vi "Set Column Width.vi"(7 "Sheet Name":string, 8 "error in":errorcluster, 9 "Width":dbl=8.43, 10 "Columns Range":string="A:C", 11 "SpreadsheetDoc":refnum<k24>) -> (0 "error out":errorcluster, 3 "SpreadsheetDoc out":refnum<k24>)   [LabVIEW 2019, in "Open Xml.lvlib"]
uses:
  Open Xml.lvlib
  D:/git/Open-Xml-LabVIEW/Source/DocumentFormat.OpenXml.dll
  DocumentFormat.OpenXml.dll
  D:/git/Open-Xml-LabVIEW/Source/DocumentFormat.OpenXml.Framework.dll
  DocumentFormat.OpenXml.Framework.dll
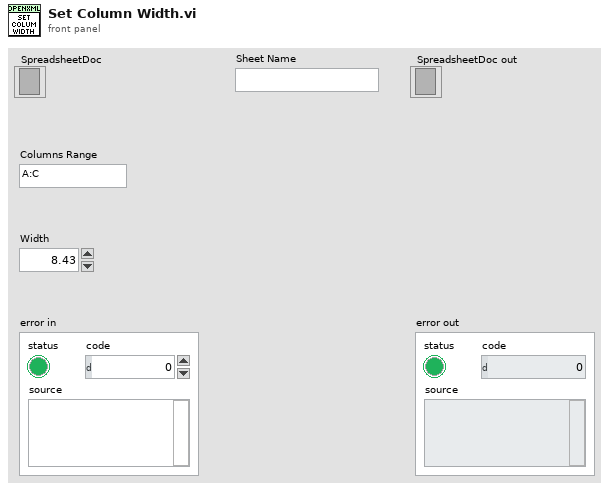
[diagram p1: front panel]
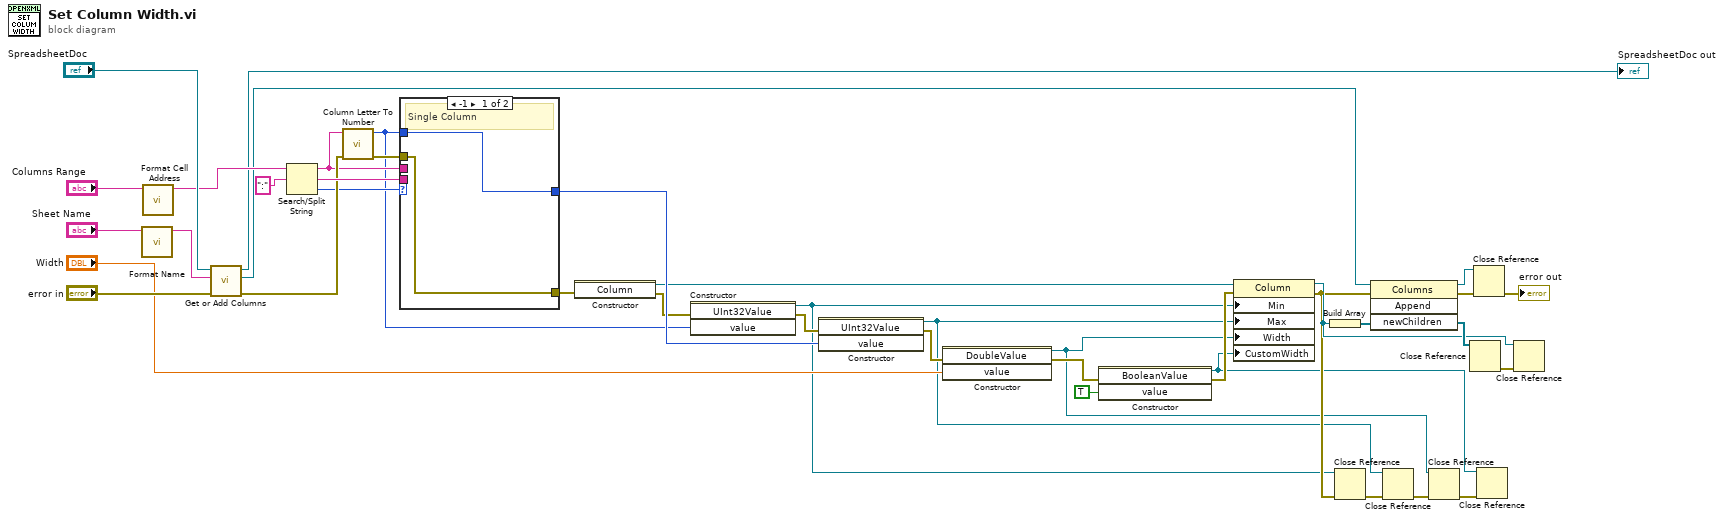
[diagram p0: block diagram]
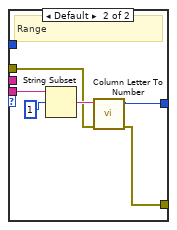
[diagram p2: hidden frame]
diagram:
  n1 = call "Format Name.vi"("Sheet Name"="Sheet Name") -> ("Formatted Sheet Name"=w37:string)  [unwired: 10 in]
  n2 = call "Format Cell Address.vi"("Cell Address"="Columns Range") -> ("Formatted Cell Address"=w35:string)  [unwired: 10 in]
  n3 = call "Get or Add Columns.vi"("error in"="error in", "Sheet Name"=w37, "SpreadsheetDoc in"="SpreadsheetDoc") -> ("error out"=w32:errorcluster, "Columns"=w17:refnum<k24>, "SpreadsheetDoc out"=→"SpreadsheetDoc out":refnum<k24>)  [unwired: 6 in]
  n4 = Search/Split String(string=w35, search string/char (-)=":") -> (substring before match=w29:string, match + rest of string=w33:string, offset of match=w31:i32)  [unwired: 1 in]
  n5 = call "Column Letter To Number.vi"("error in"=w32, "Letter"=w29) -> ("error out"=w30:errorcluster, "Number"=w18:i32)  [unwired: 8 in]
  n6 = case shown="-1" w31 {
    tunnel: w29 -> [_ _]
    tunnel: w33 -> [_ w48]
    tunnel: w30 -> [w42 w45]
    tunnel: [w42 w44] -> w21
    tunnel: [w41 w43] -> w27
    tunnel: w18 -> [w41 _]
    frame -1 {
      # "Single Column"
    }
    frame Default {
      # "Range"
      n7 = String Subset(string=w48, offset (0)=1) -> (substring=w46:string)  [unwired: 1 in]
      n8 = call "Column Letter To Number.vi"("error in"=w45, "Letter"=w46) -> ("error out"=w44:errorcluster, "Number"=w43:i32)  [unwired: 8 in]
    }
  }
  n9 = constructor class="Column"(error in=w21) -> (reference out=w19:refnum<k24>, error out=w20:errorcluster)  [unwired: 2 in, 1 out]
  n10 = constructor class="UInt32Value"(error in=w20, "value"=w18) -> (reference out=w1:refnum<k24>, error out=w28:errorcluster)  [unwired: 2 in, 2 out]
  n11 = constructor class="UInt32Value"(error in=w28, "value"=w27) -> (reference out=w2:refnum<k24>, error out=w25:errorcluster)  [unwired: 2 in, 2 out]
  n12 = constructor class="DoubleValue"(error in=w25, "value"="Width") -> (reference out=w3:refnum<k24>, error out=w24:errorcluster)  [unwired: 2 in, 2 out]
  n13 = constructor class="BooleanValue"(error in=w24, "value"=TRUE) -> (reference out=w4:refnum<k24>, error out=w22:errorcluster)  [unwired: 2 in, 2 out]
  n14 = property class="Column"(reference=w19, error in=w22, "Min"=w1, "Max"=w2, "Width"=w3, "CustomWidth"=w4) -> (reference out=w10:refnum<k24>, error out=w8:errorcluster)
  n15 = Build Array(w10) -> (w16:refnum<k24>[])
  n16 = Close Reference(reference=w1, error in (no error)=w8) -> (error out=w7:errorcluster)
  n17 = invoke class="Columns" method="Append"(reference=w17, error in=w8, "newChildren"=w16) -> (reference out=w14:refnum<k24>, error out=w15:errorcluster, "newChildren"=w11:refnum<k24>[])  [unwired: 1 in, 1 out]
  n18 = Close Reference(reference=w2, error in (no error)=w7) -> (error out=w6:errorcluster)
  n19 = Close Reference(reference=w3, error in (no error)=w6) -> (error out=w5:errorcluster)
  n20 = Close Reference(reference=w11) -> (error out=w12:errorcluster)  [unwired: 1 in]
  n21 = Close Reference(reference=w14, error in (no error)=w15) -> (error out=→"error out":errorcluster)
  n22 = Close Reference(reference=w4, error in (no error)=w5) -> ()  [unwired: 1 out]
  n23 = Close Reference(reference=w10, error in (no error)=w12) -> ()  [unwired: 1 out]
